vi "Get Test Parameters From Test Step.vi"(8 "error in (no error)":errorcluster, 9 "Test Configuration (\"\")":string, 11 "Test_ID (\"\")":string) -> (0 "error out":errorcluster, 3 "Test Parameters":variant)   [LabVIEW 2011]
uses:
  Test Function.ctl
  Test Return Parameter.ctl
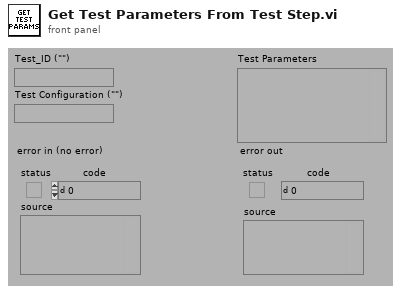
[diagram p1: front panel]
types:
  T1 = typedef "Test Function.ctl" = enum16{"Test Config", "Test Storage", "Test Pre-Process", "Unflatten Test Parameters", "Flatten Test Parameters"}
  T2 = typedef "Test Return Parameter.ctl" = enum16{"Test Parameters", "Required Instruments", "Datasheets", "QuickMode"}
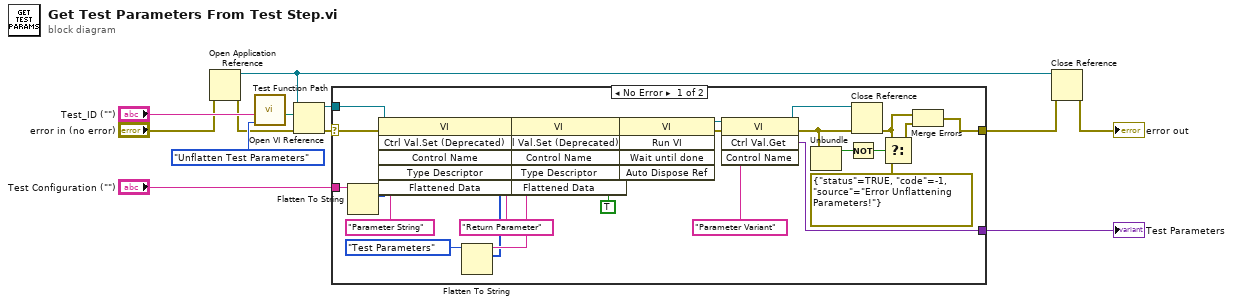
[diagram p0: block diagram]
diagram:
  n1 = Open Application Reference(8:"error in (no error)") -> (0:w1:errorcluster, 3:w3:refnum<vi>)  [unwired: 3 in]
  n2 = call "Test Function Path.vi"("Object Type (Test Config)"=Test_Function."Unflatten Test Parameters", "Object Name (\"\")"="Test_ID (\"\")") -> ("Object Path"=w8:path)  [unwired: 1 in, 8 out]
  n3 = Open VI Reference(application reference (local)=w3, vi path=w8, error in (no error)=w1) -> (vi reference=w10:refnum<vi>, error out=w11:errorcluster)  [unwired: 1 in, 2 out]
  n4 = case shown="No Error" w11 {
    selector: w11 -> [w39 w40]
    tunnel: w10 -> [w38 _]
    tunnel: "Test Configuration (\"\")" -> [w28 _]
    tunnel: [w32 w40] -> w4
    tunnel: [w13 _] -> w6
    frame No Error {
      n5 = Flatten To String(anything=w28) -> (data string=w27:string, type string=w17:i16[])  [unwired: 1 in, 3 out]
      n6 = invoke class="VI" method="Ctrl Val.Set (Deprecated)"(reference=w38, error in=w39, "Control Name"="Parameter String", "Type Descriptor"=w17, "Flattened Data"=w27) -> (reference out=w22:refnum<vi>, error out=w23:errorcluster)  [unwired: 1 in, 4 out]
      n7 = Flatten To String(anything=Test_Return_Parameter."Test Parameters" ("Return Parameter")) -> (data string=w19:string, type string=w16:i16[])  [unwired: 1 in, 3 out]
      n8 = invoke class="VI" method="Ctrl Val.Set (Deprecated)"(reference=w22, error in=w23, "Control Name"="Return Parameter", "Type Descriptor"=w16, "Flattened Data"=w19) -> (reference out=w21:refnum<vi>, error out=w20:errorcluster)  [unwired: 1 in, 4 out]
      n9 = invoke class="VI" method="Run VI"(reference=w21, error in=w20, "Wait until done"=TRUE) -> (reference out=w34:refnum<vi>, error out=w35:errorcluster)  [unwired: 2 in, 3 out]
      n10 = invoke class="VI" method="Ctrl Val.Get"(reference=w34, error in=w35, "Control Name"="Parameter Variant") -> (reference out=w33:refnum<vi>, error out=w14:errorcluster, "Get Control Value Variant"=w13:variant)  [unwired: 1 in, 1 out]
      n11 = Unbundle(w14) -> ("status"=w26:bool)  [unwired: 2 out]
      n12 = Not(x=w26) -> (.not. x?=w25:bool)
      n13 = Close Reference(reference=w33, error in (no error)=w14) -> (error out=w29:errorcluster)
      n14 = Select(t=w29, s=w25, f=errorcluster {"status"=TRUE, "code"=-1, "source"="Error Unflattening Parameters!"}) -> (s? t:f=w30:errorcluster)
      n15 = Merge Errors(w29, w30) -> (w32:errorcluster)
    }
    frame Error {
    }
  }
  "Test Parameters" <- w6
  n16 = Close Reference(reference=w3, error in (no error)=w4) -> (error out=→"error out":errorcluster)
